vi "Open Excel File (old).vi"(6 "Version (Excel 2007+)":enum16{"Excel 2007+", "Excel 2003-"}(ring), 8 "error in (no error)":errorcluster, 10 "File Name":path) -> (0 "error out":errorcluster, 3 "IWorkbook Reference Out":refnum<k24>)   [LabVIEW 2013]
uses:
  C:/PhaeronGit/LVNPOI/Resources/NPOI 2.1.1 dotnet2/NPOI.dll
  Resources/NPOI 2.1.1 dotnet2/NPOI.dll
  C:/PhaeronGit/LVNPOI/Resources/NPOI 2.1.1 dotnet4/NPOI.OOXML.dll
  Resources/NPOI 2.1.1 dotnet4/NPOI.OOXML.dll
  <vilib>/Utility/error.llb/Error Cluster From Error Code.vi
  <vilib>/ErrorRing/Error Ring.xnode
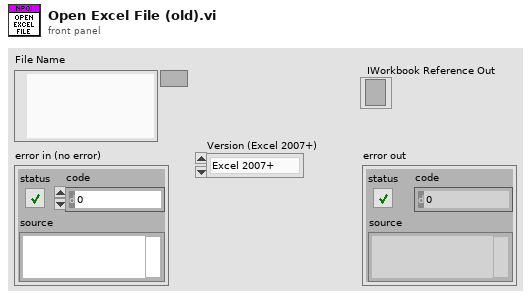
[diagram p1: front panel]
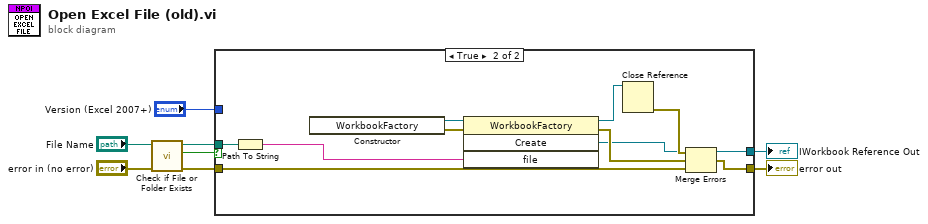
[diagram p0: block diagram]
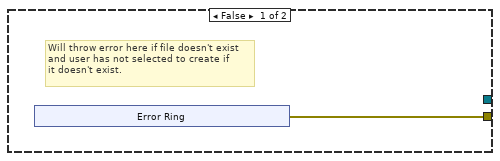
[diagram p2: hidden frame]
diagram:
  n1 = call <vilib>:"Check if File or Folder Exists.vi"("error in (no error)"="error in (no error)", "path"="File Name") -> ("error out"=w4:errorcluster, "file or folder exists?"=w3:bool, "dup path"=w5:path)  [unwired: 7 in]
  n2 = case shown="True" w3 {
    tunnel: [w9 w16] -> w8
    tunnel: w4 -> [_ w15]
    tunnel: w5 -> [_ w23]
    tunnel: "Version (Excel 2007+)" -> [_ _]
    tunnel: [_ w17] -> w1
    frame False {
      # "Will throw error here if file doesn't exist\nand user has not selected to create if\nit doesn't exist."
      n3 = xnode "Error Ring"() -> ("error out"=w9:errorcluster)
    }
    frame True {
      n4 = Path To String(path=w23) -> (string=w14:string)
      n5 = constructor class="WorkbookFactory"() -> (reference out=w18:refnum<k24>, error out=w19:errorcluster)  [unwired: 3 in, 1 out]
      n6 = invoke class="WorkbookFactory" method="Create"(reference=w18, error in=w19, "file"=w14) -> (reference out=w20:refnum<k24>, error out=w21:errorcluster, "Create"=w17:refnum<k24>)  [unwired: 1 in, 1 out]
      n7 = Close Reference(reference=w20) -> (error out=w22:errorcluster)  [unwired: 1 in]
      n8 = Merge Errors(w22, w21, w15) -> (w16:errorcluster)
    }
  }
  "IWorkbook Reference Out" <- w1
  "error out" <- w8
